vi "SVPO Scale Voltage to EU (1 Ch SGL Array).vi"(10 "channel info":T1={"sensor sensitivity"=1000.0, "engineering units"=1, "dB reference"=1.0, "custom label"="EU", "weighting filter"=0, "pregain"=0.0} {"pregain" format="%.2f"; "weighting filter" items=["Linear", "A-weighting", "B-weighting", "C-weighting", "ITU-R 468-4", "Dolby", "CCITT", "C-message", "Wb", "Wc", "Wd", "We", "Wf", "Wh", "Wj", "Wk", "Wm", "AES17 20 kHz lowpass", "AES17 40 kHz lowpass", "AES17 20 kHz highpass", "AES17 40 kHz highpass"]; "dB reference" format="%^.1e"; "engineering units" items=["custom..."=0, "V"=1, "A"=21, "C"=30, "pC"=31, "s"=32, "-"=29, "Pa"=2, "N"=20, "g"=3, "m/s^2"=4, "m/s"=5, "m"=6, "mm/s"=12, "mm"=13, "micron/s"=14, "micron"=15, "in/s^2"=7, "in/s"=8, "in"=9, "mil/s"=10, "mil"=11, "rad/s^2"=16, "rad/s"=17, "rad"=18, "deg/s^2"=26, "deg/s"=27, "deg"=28, "RPM"=22, "cycle/s^2"=23, "Hz"=24, "cycle"=25, "strain"=19]; "sensor sensitivity" format="%#_5f"}, 11 "signal [V]":sgl[](array[numeric])) -> (2 "unit label":string, 3 "scaled signal [EU]":sgl[](array[numeric]))   [LabVIEW 2017, in "SoundVib_Calibration.lvlib"]
doc: "Scales the single-precision <B>signal [V]</B> from volts to the engineering units (EU) you select. Scale signals to appropriate EU before applying limits, saving to disk, and performing measurement analyses. Use this VI on embedded targets that have limited computational resources. Wire data to the <B>signal [V]</B> input to determine the polymorphic instance to use or manually select the instance."
uses:
  <vilib>/addons/Sound and Vibration/svt_Calibration/SoundVib_Calibration.lvlib
  <vilib>/addons/_NISVFA/_Shared subVIs/Controls/svc_Channel Info.ctl
  <vilib>/addons/_NISVFA/_Shared subVIs/Controls/svc_Engineering Units Text Ring.ctl
  <vilib>/addons/_NISVFA/_Shared subVIs/Controls/svc_Weighting Filter Text Ring.ctl
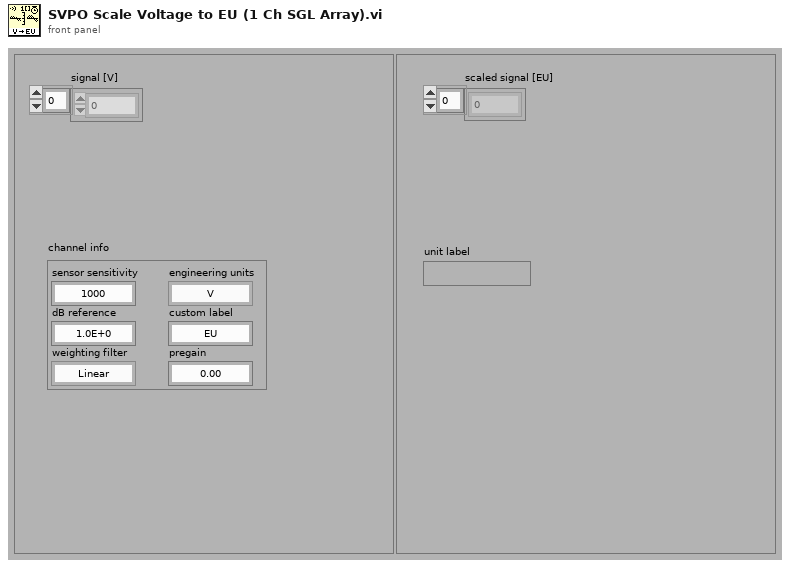
[diagram p1: front panel]
types:
  T1 = typedef "svc_Channel Info.ctl" = cluster{"sensor sensitivity":dbl, "engineering units":T2, "dB reference":dbl, "custom label":string, "weighting filter":T3, "pregain":dbl}
  T2 = typedef "svc_Engineering Units Text Ring.ctl" = u16
  T3 = typedef "svc_Weighting Filter Text Ring.ctl" = u16
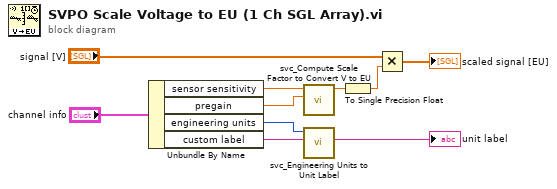
[diagram p0: block diagram]
diagram:
  n1 = Unbundle By Name("channel info") -> ("sensor sensitivity"=w1:dbl, "pregain"=w7:dbl, "engineering units"=w6:T2, "custom label"=w5:string)
  n2 = call <vilib>:"svc_Compute Scale Factor to Convert V to EU.vi"("pregain [dB]"=w7, "sensor sensitivity [mV/EU]"=w1) -> ("EU scale factor [EU/V]"=w3:dbl)  [unwired: 9 in]
  n3 = call <vilib>:"svc_Engineering Units to Unit Label.vi"("custom label"=w5, "engineering units"=w6) -> ("unit label"=→"unit label":string)  [unwired: 8 in, 1 out]
  n4 = To Single Precision Float(number=w3) -> (single precision float=w9:sgl)
  n5 = Multiply(x="signal [V]", y=w9) -> (x*y=→"scaled signal [EU]":sgl[])
